vi "Extract Print Line.vi"(11 "data value reference":refnum<data-value>) -> (1 "End of Print?":bool=TRUE, 2 "Current Line":T1, 3 "data value reference":refnum<data-value>)   [LabVIEW 2018, in "Stage Actor.lvlib"]
uses:
  Stage Actor.lvlib
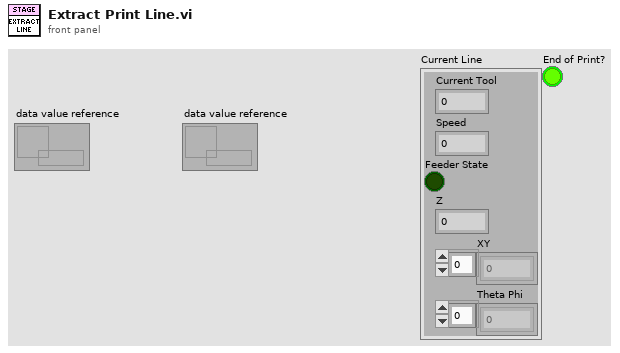
[diagram p1: front panel]
types:
  T1 = cluster{"Current Tool":i16, "Speed":dbl, "Feeder State":bool, "Z":dbl, "XY":dbl[], "Theta Phi":dbl[]}
  T2 = cluster{"XY":dbl[][], "Theta Phi":dbl[][], "Current Tool":i16[], "Speed":dbl[], "Feeder State":bool[], "Z":dbl[]}
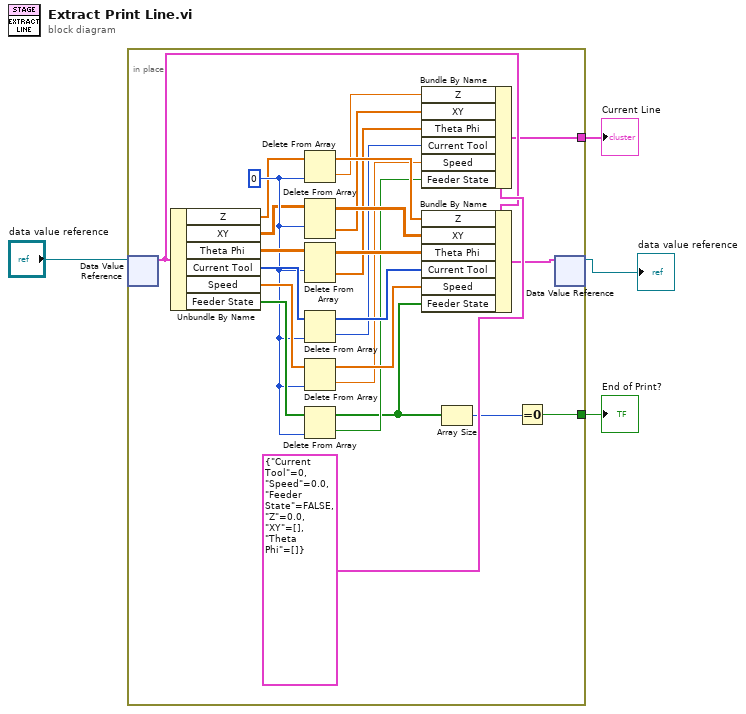
[diagram p0: block diagram]
diagram:
  n1 = in-place {
    in-place-border: [w7] -> w3
    in-place-border: [w5] -> w2
    w25 = 0
    n2 = in-place-dvr #1("data value reference") -> (w8:T2)  [unwired: 1 out]
    n3 = Unbundle By Name(w8) -> ("Z"=w24:dbl[], "XY"=w23:dbl[][], "Theta Phi"=w29:dbl[][], "Current Tool"=w28:i16[], "Speed"=w27:dbl[], "Feeder State"=w26:bool[])
    n4 = Delete From Array(array=w24, index=w25) -> (deleted portion=w17:dbl, array with subset deleted=w18:dbl[])  [unwired: 1 in]
    n5 = Delete From Array(array=w23, index (row)=w25) -> (deleted portion=w16:dbl[], array with subset deleted=w19:dbl[][])  [unwired: 2 in]
    n6 = Delete From Array(array=w29, index (row)=w25) -> (deleted portion=w15:dbl[], array with subset deleted=w20:dbl[][])  [unwired: 2 in]
    n7 = Delete From Array(array=w28, index=w25) -> (deleted portion=w14:i16, array with subset deleted=w21:i16[])  [unwired: 1 in]
    n8 = Delete From Array(array=w27, index=w25) -> (deleted portion=w13:dbl, array with subset deleted=w22:dbl[])  [unwired: 1 in]
    n9 = Delete From Array(array=w26, index=w25) -> (deleted portion=w12:bool, array with subset deleted=w9:bool[])  [unwired: 1 in]
    n10 = Bundle By Name(cluster=T1 {"Current Tool"=0, "Speed"=0.0, "Feeder State"=FALSE, "Z"=0.0, "XY"=[], "Theta Phi"=[]} ("Print Data 2"), "Z"=w17, "XY"=w16, "Theta Phi"=w15, "Current Tool"=w14, "Speed"=w13, "Feeder State"=w12) -> (w7:T1)
    n11 = Bundle By Name(cluster=w8, "Z"=w18, "XY"=w19, "Theta Phi"=w20, "Current Tool"=w21, "Speed"=w22, "Feeder State"=w9) -> (w6:T2)
    n12 = Array Size(array=w9) -> (size(s)=w10:i32)
    n13 = Equal To 0?(x=w10) -> (x = 0?=w5:bool)
    n14 = in-place-dvr #1(w6) -> (→"data value reference":refnum<data-value>)  [unwired: 1 out]
  }
  "Current Line" <- w3
  "End of Print?" <- w2
